vi "ChooseKeeperPlay.vi"(8 "error in (no error)":errorcluster, 10 "GameRef":refnum<data-value>, 11 "Playbook_v2 in":refnum<class "Playbook_v2.lvclass">) -> (0 "error out":errorcluster, 3 "Playbook_v2 out":refnum<class "Playbook_v2.lvclass">)   [LabVIEW 2023, in "Playbook_v2.lvclass"]
uses:
  Playbook_v2.lvclass
  Game_class/Game.lvclass
  NewPlays/Play_v2_class/Play_v2.lvclass
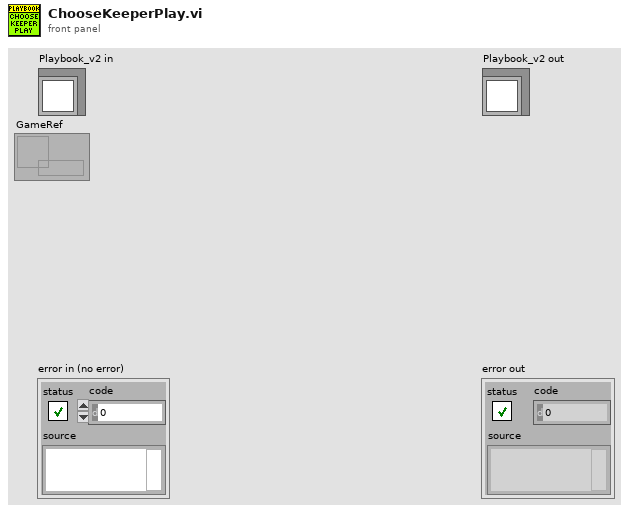
[diagram p1: front panel]
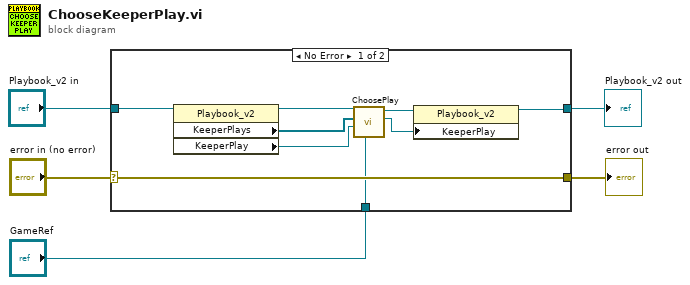
[diagram p0: block diagram]
diagram:
  n1 = case shown="No Error" "error in (no error)" {
    selector: "error in (no error)" -> [w14 w16]
    tunnel: [w14 w16] -> w4
    tunnel: [w7 w15] -> w2
    tunnel: "Playbook_v2 in" -> [w13 w15]
    tunnel: "GameRef" -> [w6 _]
    frame No Error {
      n2 = property class="Playbook_v2"(reference=w13) -> (reference out=w12:refnum<class "Playbook_v2.lvclass">, "KeeperPlays"=w11:refnum<class "Play_v2.lvclass">[], "KeeperPlay"=w10:refnum<class "Play_v2.lvclass">)  [unwired: 1 in, 1 out]
      n3 = call "ChoosePlay.vi"("GameRef"=w6, "currentPlay"=w10, "plays"=w11, "Playbook_v2 in"=w12) -> ("newPlay"=w8:refnum<class "Play_v2.lvclass">, "Playbook_v2 out"=w9:refnum<class "Playbook_v2.lvclass">)  [unwired: 5 in, 1 out]
      n4 = property class="Playbook_v2"(reference=w9, "KeeperPlay"=w8) -> (reference out=w7:refnum<class "Playbook_v2.lvclass">)  [unwired: 1 in, 1 out]
    }
    frame Error {
    }
  }
  "error out" <- w4
  "Playbook_v2 out" <- w2
